vi "Disable Analysis Workspace.vi"(8 "error in (no error)":errorcluster) -> (0 "error out":errorcluster)   [LabVIEW 2018, in "NI_AALPro.lvlib"]
doc: "Disables the use of the analysis workspace. To prevent race conditions, priority inversions, and other undefined behavior, you must use the Disable Analysis Workspace VI according to a strict set of guidelines."
uses:
  <vilib>/Analysis/NI_AALPro.lvlib
  <resource>/lvanlys.dll
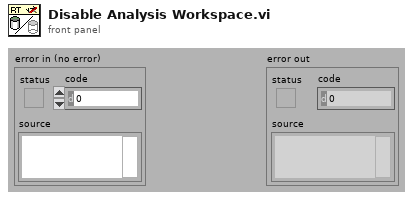
[diagram p1: front panel]
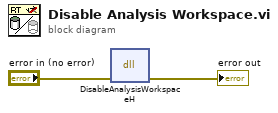
[diagram p0: block diagram]
diagram:
  n1 = dll-call lib="C:/Program Files (x86)/National Instruments/LabVIEW 2018/resource/lvanlys.*" fn="DisableAnalysisWorkspaceH"("_errorCluster"="error in (no error)") -> ("_errorCluster"=→"error out":errorcluster)  [unwired: 4 in, 2 out]
